vi "Window_SQL_Services.vi"() -> ()   [LabVIEW 2017]
uses:
  System.ServiceProcess
panel:
  out "Array":string[](array[string])
  out "Status":i32[](array[ring]) items=["Stopped"=1, "StartPending"=2, "StopPending"=3, "Running"=4, "ContinuePending"=5, "PausePending"=6, "Paused"=7]
  in  "error in":errorcluster
  out "error out":errorcluster
  in  "reference":refnum<k24>
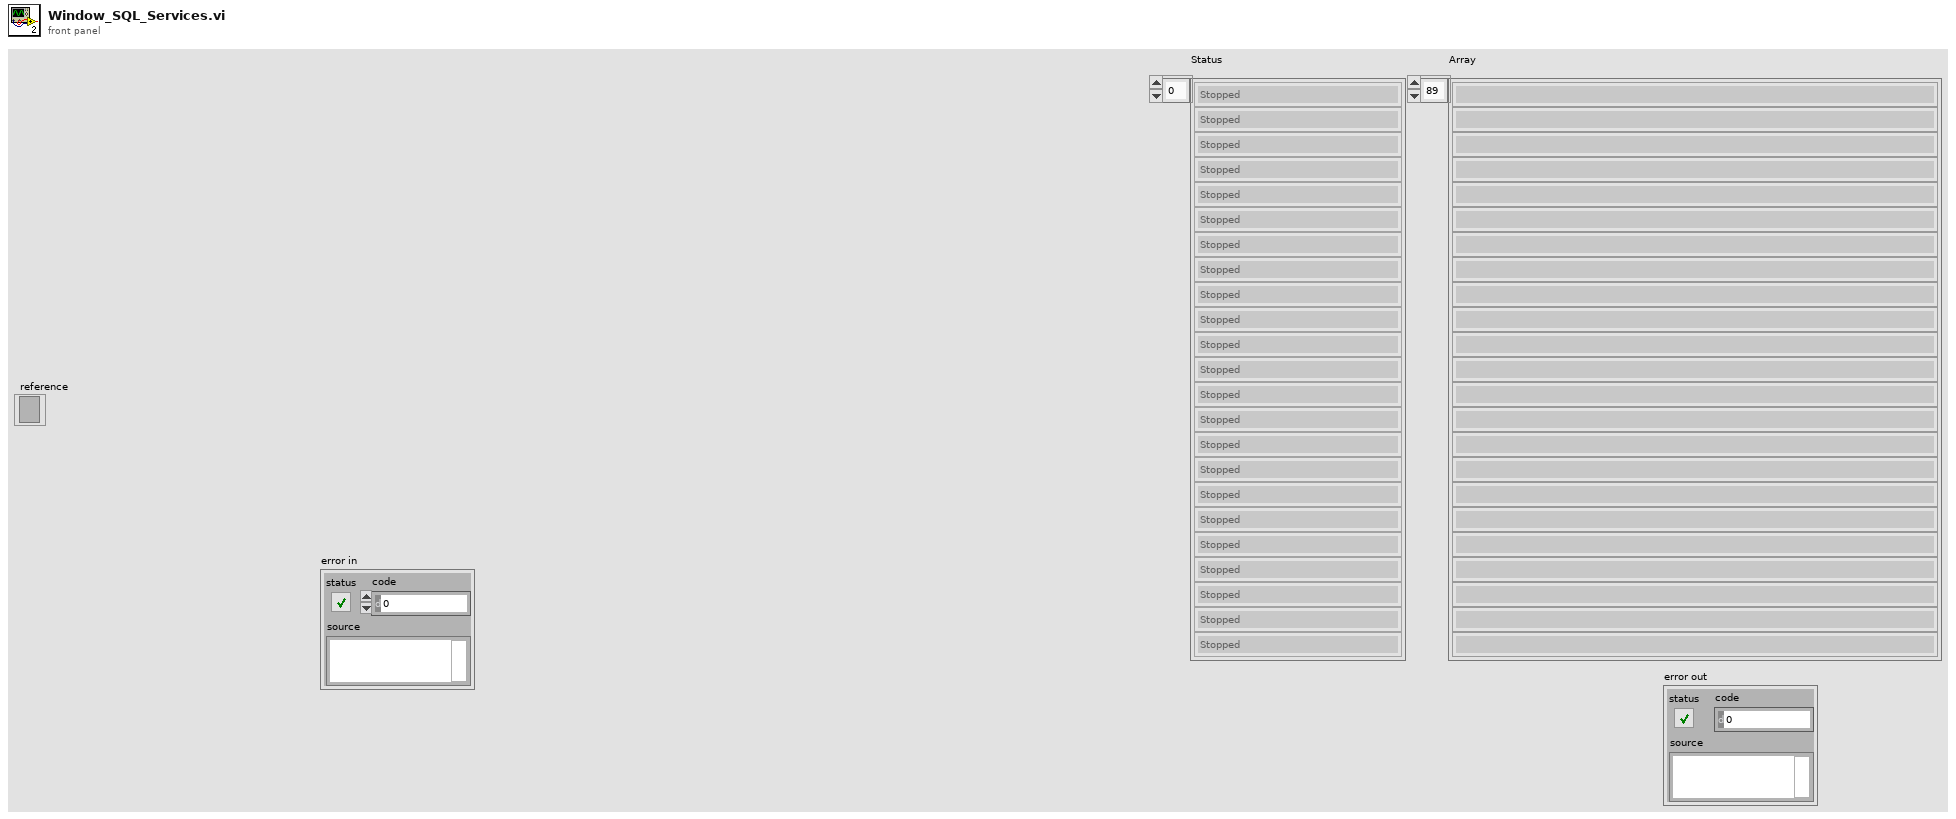
[diagram p1: front panel]
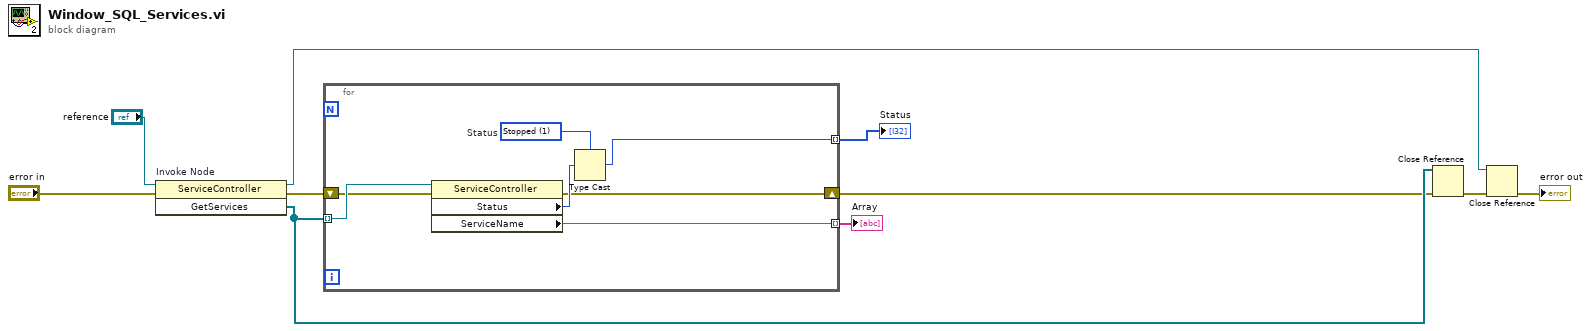
[diagram p0: block diagram]
diagram:
  n1 = invoke on="Invoke Node" class="ServiceController" method="GetServices"(reference="reference", error in="error in") -> (reference out=w4:refnum<k24>, error out=w9:errorcluster, "GetServices"=w6:refnum<k24>[])  [unwired: 1 in]
  n2 = for {
    tunnel: w6 -> [w17] mode=indexing
    tunnel: [w14] -> w2 mode=indexing
    shift-right: [w12] -> w5
    shift-left: w9 -> [w13]
    tunnel: [w11] -> w1 mode=indexing
    w16 = 1 items=["Stopped"=1, "StartPending"=2, "StopPending"=3, "Running"=4, "ContinuePending"=5, "PausePending"=6, "Paused"=7]  # Status
    n3 = property class="ServiceController"(reference=w17, error in=w13) -> (error out=w12:errorcluster, "Status"=w15:i32, "ServiceName"=w11:string)  [unwired: 1 out]
    n4 = Type Cast(type=w16, x=w15) -> (*(type *) &x=w14:i32)
  }
  "Status" <- w2
  "Array" <- w1
  n5 = Close Reference(reference=w6, error in (no error)=w5) -> (error out=w8:errorcluster)
  n6 = Close Reference(reference=w4, error in (no error)=w8) -> (error out=→"error out":errorcluster)
